vi "activationError.vi"(8 "error in (no error)":errorcluster, 10 "DeviceId":u8[](array[numeric]), 11 "SEDSpectrometer in":refnum<class "SEDSpectrometer.lvclass">) -> (0 "error out":errorcluster, 2 "Status":string, 3 "SEDSpectrometer out":refnum<class "SEDSpectrometer.lvclass">)   [LabVIEW 2016, in "SEDSpectrometer.lvclass"]
uses:
  SEDSpectrometer.lvclass
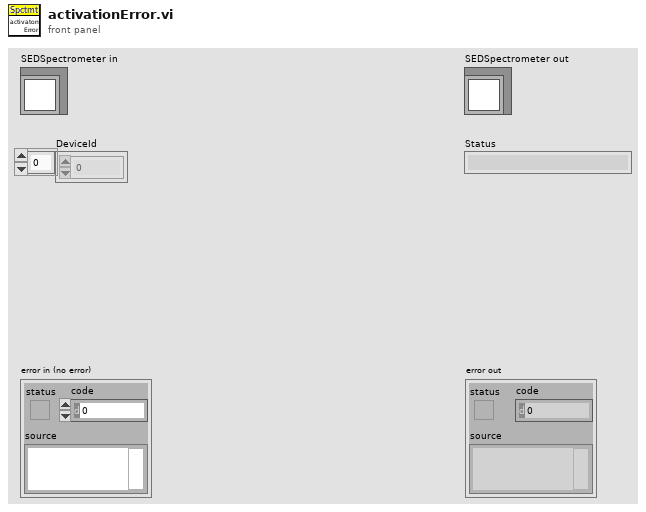
[diagram p1: front panel]
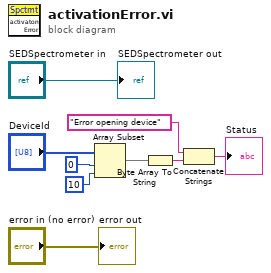
[diagram p0: block diagram]
diagram:
  n1 = Array Subset(array="DeviceId", index=0 ("length"), length=10) -> (w1:u8[])
  n2 = Byte Array To String(unsigned byte array=w1) -> (string=w5:string)
  n3 = Concatenate Strings("Error opening device", w5) -> (→"Status":string)
  "error out" <- "error in (no error)"
  "SEDSpectrometer out" <- "SEDSpectrometer in"
